vi "Example2.vi"() -> ()   [LabVIEW 2019]
panel:
  in  "K":dbl
  out "J":dbl
  in  "I":dbl
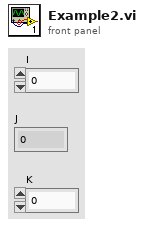
[diagram p1: front panel]
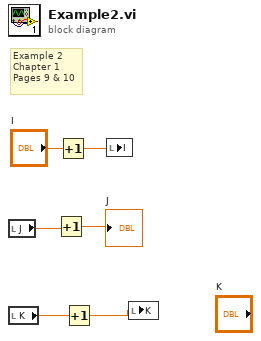
[diagram p0: block diagram]
diagram:
  # "Example 2 \nChapter 1\nPages 9 & 10"
  n1 = local read "J"() -> (w3:dbl)
  n2 = local read "K"() -> (w2:dbl)
  n3 = Increment(x=w3) -> (x+1=→"J":dbl)
  n4 = Increment(x="I") -> (x+1=w5:dbl)
  n5 = Increment(x=w2) -> (x+1=w1:dbl)
  n6 = local write "I"(w5) -> ()
  n7 = local write "K"(w1) -> ()
